vi "create.vi"(0 "MIILCFactory in":refnum<class "MIILCFactory.lvclass">, 5 "MISettings":T3, 7 "ILCTimings":T1, 9 "MITimings":T2, 11 "error in (no error)":errorcluster) -> (4 "MIILCFactory out":refnum<class "MIILCFactory.lvclass">, 6 "MIILC":refnum<class "MIILC.lvclass">, 15 "error out":errorcluster)   [LabVIEW 2016, in "RTMIILC.lvlib" / "MIILCFactory.lvclass"]
uses:
  MIILCFactory.lvclass
  DataTypes/MISettings.ctl
  Common_RT_ILC/DataTypes/ILCSettings.ctl
  MIILC/MIILC.lvclass
  D:/Code/Common_RT_ILC/ILC/ILC.lvclass
  DataTypes/MITimings.ctl
  Common_RT_ILC/DataTypes/ILCTimings.ctl
  Common_RT_ILC/ILCFactory/ILCFactory.lvclass
  DataTypes/MIData.ctl
  DataTypes/MIConstants.ctl
  DataTypes/MITelemetry.ctl
  DataTypes/MIResponses.ctl
  Common_RT_Modbus/DataTypes/ExceptionCodes.ctl
  MIILC/MIILC.lvclass/MIILC.ctl
  RTMIILC.lvlib
  Common_RT_Modbus/RTModbus.lvlib
  Common_RT_ILC/RTILC.lvlib
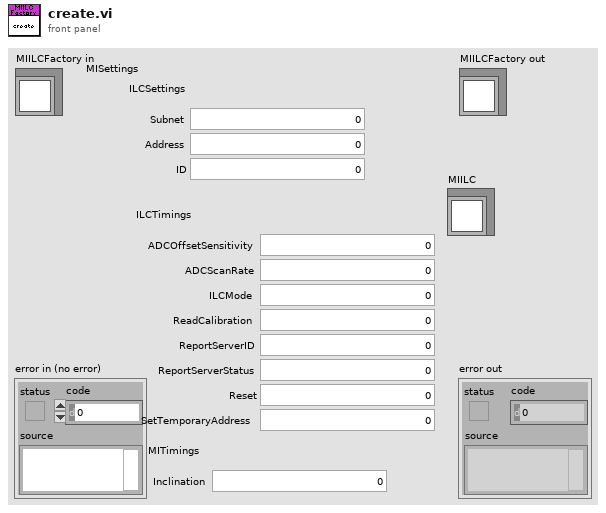
[diagram p1: front panel]
types:
  T1 = typedef "RTILC.lvlib/ILCTimings.ctl" = cluster{"ADCOffsetSensitivity":u32, "ADCScanRate":u32, "ILCMode":u32, "ReadCalibration":u32, "ReportServerID":u32, "ReportServerStatus":u32, "Reset":u32, "SetTemporaryAddress":u32}
  T2 = typedef "RTMIILC.lvlib/MITimings.ctl" = cluster{"Inclination":u32}
  T3 = typedef "RTMIILC.lvlib/MISettings.ctl" = cluster{"ILCSettings":T4, "ID":i16}
  T4 = typedef "RTILC.lvlib/ILCSettings.ctl" = cluster{"Subnet":u8, "Address":u8}
  T5 = typedef "RTMIILC.lvlib/MIData.ctl" = cluster{"Constants":T6, "Telemetry":T7, "Responses":T8, "Timings":T2}
  T6 = typedef "RTMIILC.lvlib/MIConstants.ctl" = cluster{"ID":i16}
  T7 = typedef "RTMIILC.lvlib/MITelemetry.ctl" = cluster{"Angle":sgl}
  T8 = typedef "RTMIILC.lvlib/MIResponses.ctl" = cluster{"Inclination":T9}
  T9 = typedef "RTModbus.lvlib/ExceptionCodes.ctl" = u16
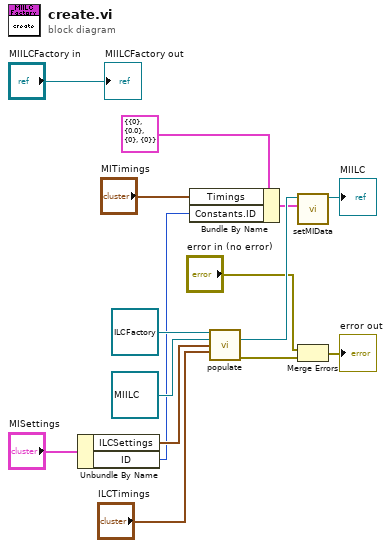
[diagram p0: block diagram]
diagram:
  n1 = Unbundle By Name("MISettings") -> ("ILCSettings"=w14:T4, "ID"=w9:i16)
  n2 = Bundle By Name(cluster=T5 {"Constants"={"ID"=0}, "Telemetry"={"Angle"=0.0}, "Responses"={"Inclination"=0}, "Timings"={"Inclination"=0}} ("MTData"), "Timings"="MITimings", "Constants.ID"=w9) -> (w8:T5)
  n3 = call "populate.vi"("ILCFactory in"=refnum<class "ILCFactory.lvclass"> refnum ("RTILC.lvlib:ILCFactory.lvclass"), "ILC in"=refnum<class "MIILC.lvclass"> refnum ("RTMTILC.lvlib:MTILC.lvclass"), "Settings"=w14, "Timings"="ILCTimings") -> ("ILC out"=w11:refnum<class "MIILC.lvclass">, "error out"=w6:errorcluster)  [unwired: 9 in, 1 out]
  n4 = call "setMIData.vi"("MIData"=w8, "MIILC in"=w11) -> ("MIILC out"=→"MIILC":refnum<class "MIILC.lvclass">)  [unwired: 9 in]
  n5 = Merge Errors("error in (no error)", w6) -> (→"error out":errorcluster)
  "MIILCFactory out" <- "MIILCFactory in"
